vi "swap data buffers.vi"(3 "sink queue":refnum<queue>, 8 "error in":errorcluster, 10 "data table in":T1, 11 "source queue":refnum<queue>) -> (0 "error out":errorcluster, 2 "data table out":T1)   [LabVIEW 2013, in "Standard Engine Runtime.lvclass"]
uses:
  Standard Engine Runtime.lvclass
  <vilib>/NI/Tag Bus/table/data table.ctl
  <vilib>/NI/Tag Bus/table/data table.lvlib
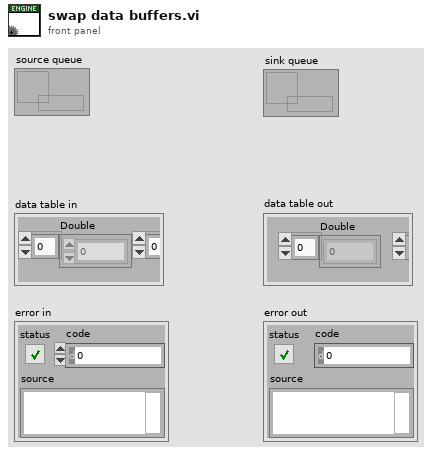
[diagram p1: front panel]
types:
  T1 = typedef "tag bus.lvlib/data table.lvlib/data table.ctl" = cluster{"Double":dbl[], "Single":sgl[], "I64":i64[], "I32":i32[], "I16":i16[], "I8":i8[], "U64":u64[], "U32":u32[], "U16":u16[], "U8":u8[], "Boolean":bool[], "String":string[], "Array of Double":cluster{"DBL Array":dbl[]}[], "Array of Single":cluster{"SGL Array":sgl[]}[], "Array of I64":cluster{"I64 Array":i64[]}[], "Array of I32":cluster{"I32 Array":i32[]}[], "Array of I16":cluster{"I16 Array":i16[]}[], "Array of I8":cluster{"I8 Array":i8[]}[], "Array of U64":cluster{"U64 Array":u64[]}[], "Array of U32":cluster{"U32 Array":u32[]}[], "Array of U16":cluster{"U16 Array":u16[]}[], "Array of U8":cluster{"U8 Array":u8[]}[], "Array of Boolean":cluster{"Boolean Array":bool[]}[], "Array of String":cluster{"String Array":string[]}[]}
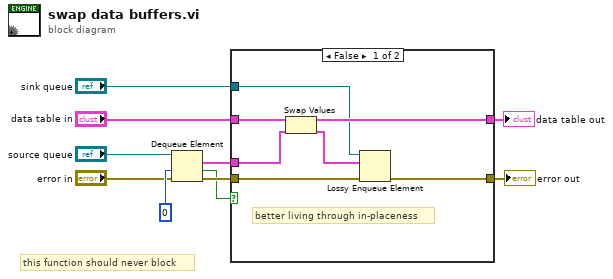
[diagram p0: block diagram]
diagram:
  # "this function should never block"
  n1 = Dequeue Element(queue="source queue", timeout in ms (-1)=0, error in (no error)="error in") -> (element=w10:T1, timed out?=w7:bool, error out=w8:errorcluster)  [unwired: 1 out]
  n2 = case shown="False" w7 {
    tunnel: w8 -> [w13 w19]
    tunnel: [w17 w19] -> w9
    tunnel: "data table in" -> [w16 w18]
    tunnel: [w14 w18] -> w1
    tunnel: w10 -> [w15 _]
    tunnel: "sink queue" -> [w11 _]
    frame False {
      # "better living through in-placeness"
      n3 = Swap Values(12:w16, 14:w15) -> (1:w14:T1, 3:w12:T1)  [unwired: 1 in]
      n4 = Lossy Enqueue Element(queue=w11, element=w12, error in (no error)=w13) -> (error out=w17:errorcluster)  [unwired: 3 out]
    }
    frame True {
    }
  }
  "error out" <- w9
  "data table out" <- w1
